vi "test_Multiple Local Comparison Response Messages using Trigger.vi"(8 "error in (no error)":errorcluster, 11 "TestCase in":refnum<class "Common System Tests.lvclass">) -> (0 "error out":errorcluster, 3 "TestCase out":refnum<class "Common System Tests.lvclass">)   [LabVIEW 2018, in "Common System Tests.lvclass"]
uses:
  Common System Tests.lvclass
  C:/Dev/niveristand-custom-device-testing-tools/VeriStandTestCase/VeriStandTestCase.lvclass
  <vilib>/NI Veristand/Execution/Workspace/NI VeriStand - Set Multiple Channel Values.vi
  <vilib>/NI Veristand/Execution/Workspace/NI VeriStand - Get Multiple Channel Values.vi
  <vilib>/addons/_JKI Toolkits/VI Tester/TestCase.llb/TestCase.lvclass
  <vilib>/NI Veristand/Execution/Workspace/NI_VS Workspace ExecutionAPI.lvlib
  C:/Program Files (x86)/National Instruments/LabVIEW 2018/vi.lib/addons/_JKI Toolkits/VI Tester/TestCase.llb/TestCase.lvclass
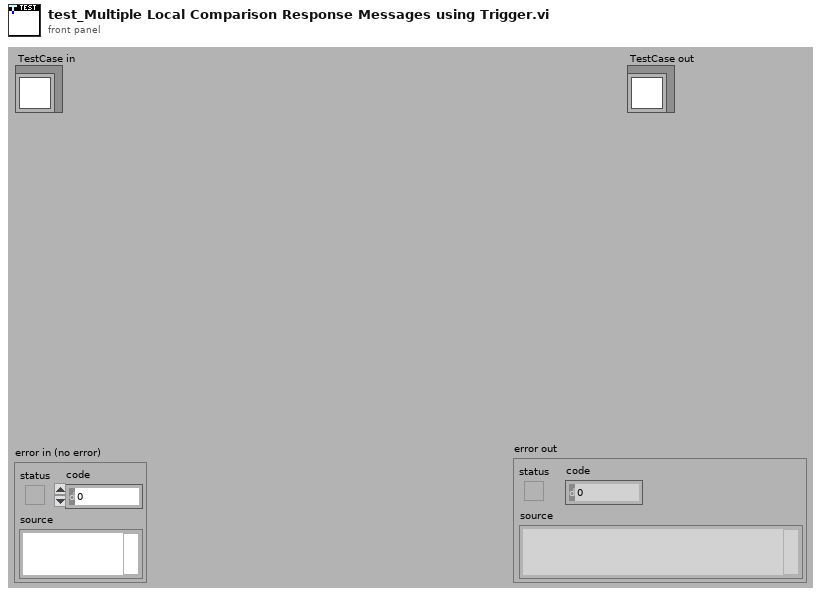
[diagram p1: front panel]
types:
  T1 = typedef "NI_VS Workspace ExecutionAPI.lvlib/WorkspaceAPI.ctl" = refnum<k24>
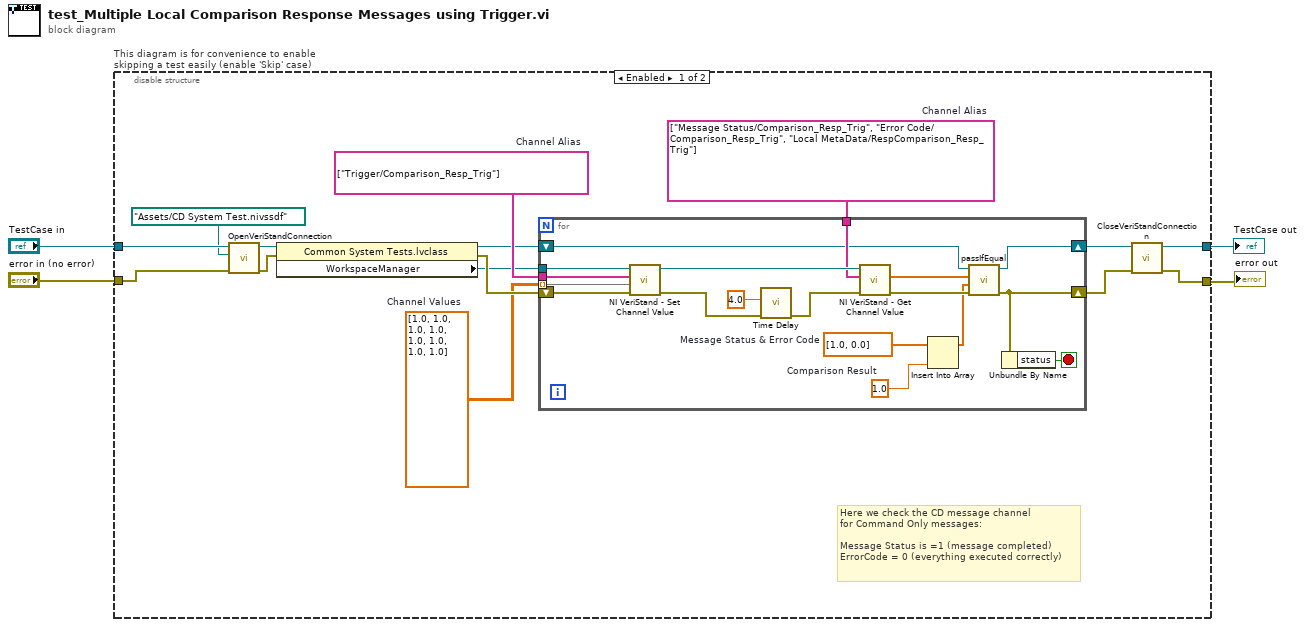
[diagram p0: block diagram]
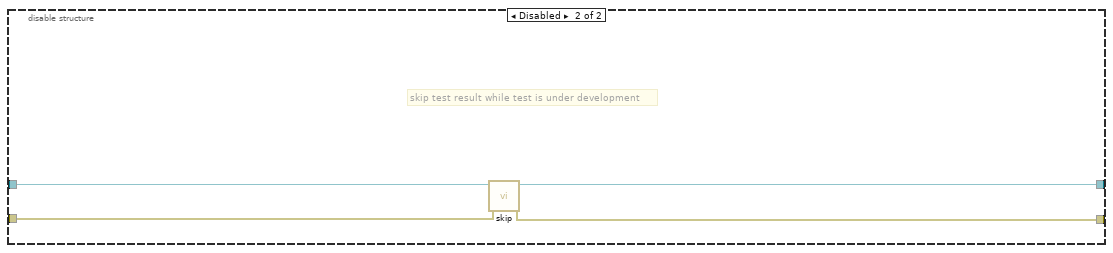
[diagram p2: hidden frame]
diagram:
  n1 = disable-structure "This diagram is for convenience to enable skipping a test easily (enable 'Skip' case)" shown="Enabled" {
    disable-tunnel: "TestCase in" -> [w17 w41]
    disable-tunnel: [w18 w39] -> w1
    disable-tunnel: [w19 w40] -> w3
    disable-tunnel: "error in (no error)" -> [w15 w38]
    frame Enabled {
      w8 = string[] ["Message Status/Comparison_Resp_Trig", "Error Code/Comparison_Resp_Trig", "Local MetaData/RespComparison_Resp_Trig"]  # Channel Alias
      w10 = dbl[][] [[1.0], [1.0], [1.0], [1.0], [1.0], [1.0], [1.0], [1.0]]  # Channel Values
      w11 = string[] ["Trigger/Comparison_Resp_Trig"]  # Channel Alias
      # "Here we check the CD message channel\nfor Command Only messages:\n\nMessage Status is =1 (message completed)\nErrorCode = 0 (everything executed correctly)"
      n2 = call-dynamic "OpenVeriStandConnection.vi"("error in (no error)"=w15, "System Definition File"=path "Assets/CD System Test.nivssdf", "VeriStand Test Case in"=w17) -> ("error out"=w14:errorcluster, "VeriStand Test Case out"=w16:refnum<class "Common System Tests.lvclass">)  [unwired: 6 in, 1 out]
      n3 = property class="Common System Tests.lvclass"(reference=w16, error in=w14) -> (reference out=w9:refnum<class "Common System Tests.lvclass">, error out=w12:errorcluster, "WorkspaceManager"=w7:T1)
      n4 = for {
        tunnel: w7 -> [w37]
        tunnel: w11 -> [w35]
        tunnel: w10 -> [w23] mode=indexing
        shift-right: [w22] -> w5
        shift-left: w12 -> [w36]
        tunnel: w8 -> [w33]
        shift-right: [w28] -> w6
        shift-left: w9 -> [w29]
        stop <- w25 stop-if-true
        w20 = 1.0  # Comparison Result
        w24 = dbl[] [1.0, 0.0]  # Message Status & Error Code
        n5 = call-poly <vilib>:"NI VeriStand - Set Channel Value.vi"("error in (no error)"=w36, "Values"=w23, "Channels"=w35, "WorkspaceManager in"=w37) -> ("error out"=w31:errorcluster, "WorkspaceManager out"=w34:T1)  [unwired: 6 in]
        n6 = call "Time Delay"("error in (no error)"=w31, "Delay Time (s)"=4.0) -> ("error out"=w30:errorcluster)  [unwired: 9 in]
        n7 = call-poly <vilib>:"NI VeriStand - Get Channel Value.vi"("error in (no error)"=w30, "Channels"=w33, "WorkspaceManager in"=w34) -> ("error out"=w27:errorcluster, "Values"=w26:dbl[])  [unwired: 6 in, 1 out]
        n8 = Insert Into Array(array=w24, new element=w20) -> (w21:dbl[])  [unwired: 1 in]
        n9 = call-dynamic "passIfEqual.vi"("error in (no error)"=w27, "y"=w21, "x"=w26, "TestCase in"=w29) -> ("error out"=w22:errorcluster, "TestCase out"=w28:refnum<class "Common System Tests.lvclass">)  [unwired: 6 in]
        n10 = Unbundle By Name(w22) -> ("status"=w25:bool)
      }
      n11 = call-dynamic "CloseVeriStandConnection.vi"("error in (no error)"=w5, "VeriStand Test Case in"=w6) -> ("error out"=w19:errorcluster, "VeriStand Test Case out"=w18:refnum<class "Common System Tests.lvclass">)  [unwired: 8 in]
    }
    frame Disabled {
      # "skip test result while test is under development"
      n12 = call <vilib>:"skip.vi"("error in (no error)"=w38, "TestCase in"=w41) -> ("error out"=w40:errorcluster, "TestCase out"=w39:refnum<class "Common System Tests.lvclass">)  [unwired: 8 in]
    }
  }
  "error out" <- w3
  "TestCase out" <- w1
